vi "04_co_dela_necelistvy_pocet_period.vi"() -> ()   [LabVIEW 2019]
uses:
  <vilib>/Analysis/5stat.llb/RMS (DBL).vi
  <vilib>/measure/NI_MABase.lvlib
  <vilib>/Analysis/NI_AALPro.lvlib
panel:
  out "Spektra":T1(graph)
  out "Absolutni chyba (V)":dbl
  out "Relativni chyba (%)":dbl
  out "RMS prubehy":cluster{dbl, dbl, dbl, dbl}(graph)
  out "RMS (V)":dbl
  out "RMS (V)":dbl
  out "RMS (mat funkce) (V)":dbl format="%0.2f"
  out "RMS (mat funkce) (V)":dbl format="%0.2f"
  out "Casove prubehy":waveform(dbl)[](graph)
  out "dt (s)":dbl=0.001
  out "Vzorkovaci Frekvence (N)":dbl=1000.0
  in  "Amplituda sumu":dbl=0.9999999999999999 format="%.2p"
  in  "Faze":dbl format="%.2p"
  in  "Amplituda":dbl=10.0 format="%0.2p"
  in  "Frekvence":dbl=10.0 format="%0.2p"
  # "CELISTVY POCET PERIOD"
  # "NECELISTVY POCET PERIOD"
  # "SLEDUJTE\nJAK SE \nCHOVAJI\nJEDNOTLIVE\nVYPOCTY !"
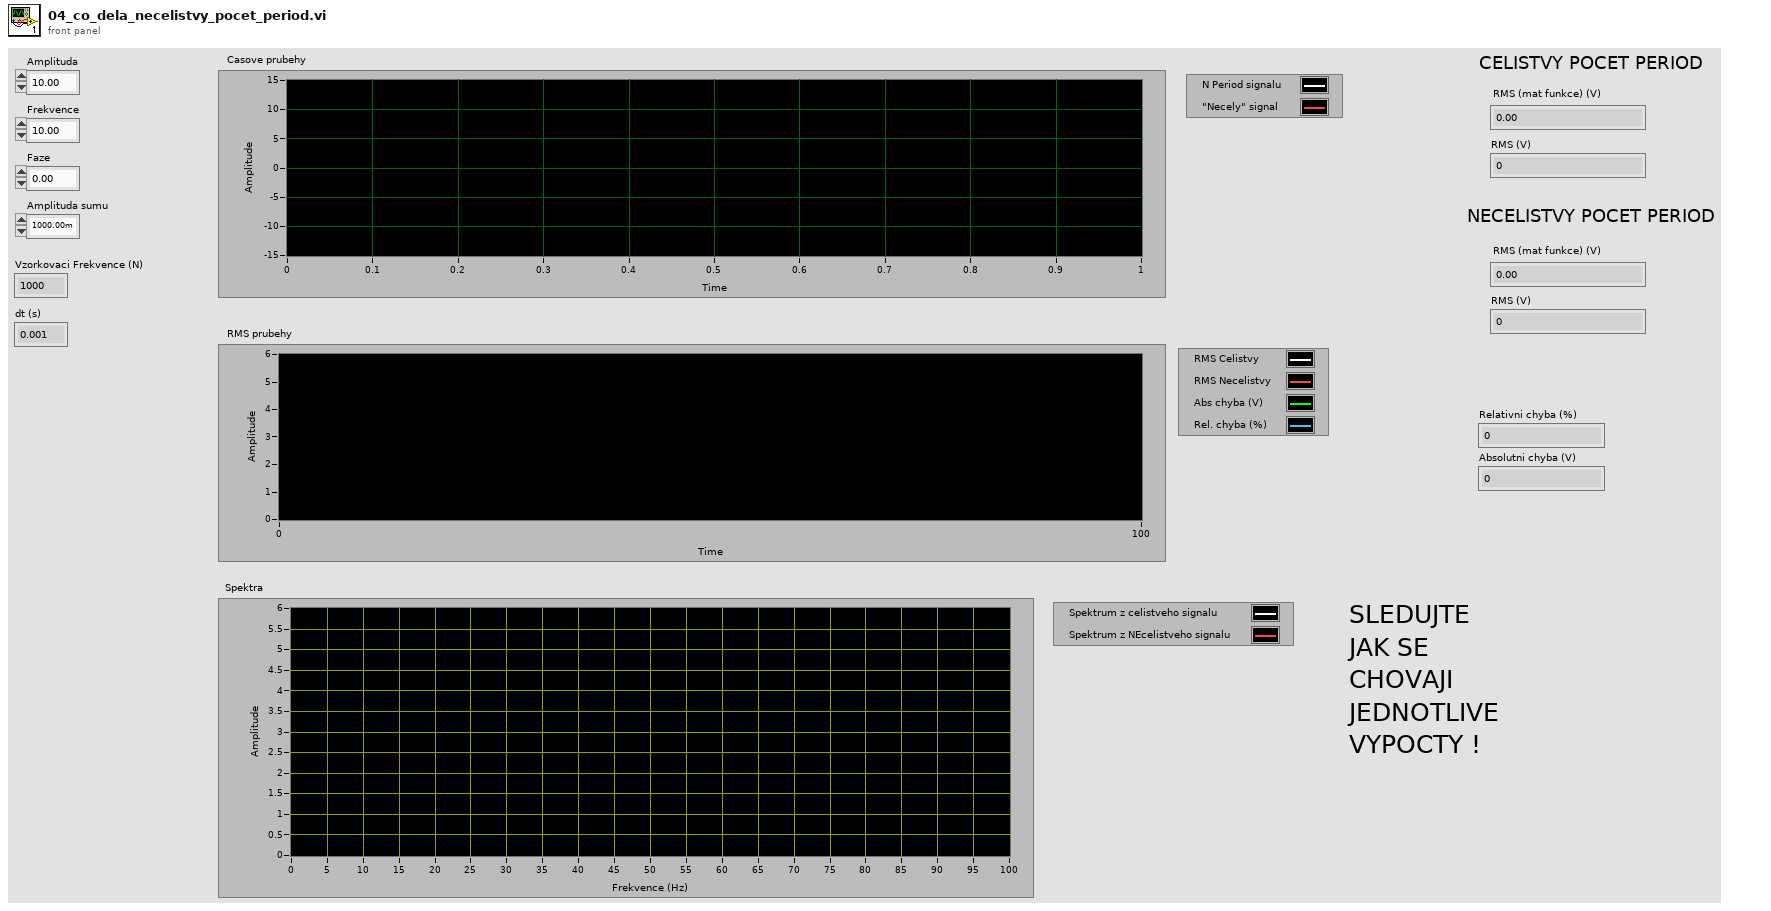
[diagram p1: front panel]
types:
  T1 = cluster{dbl[], "Amp Spectrum Mag (Vrms)":dbl[]}[]
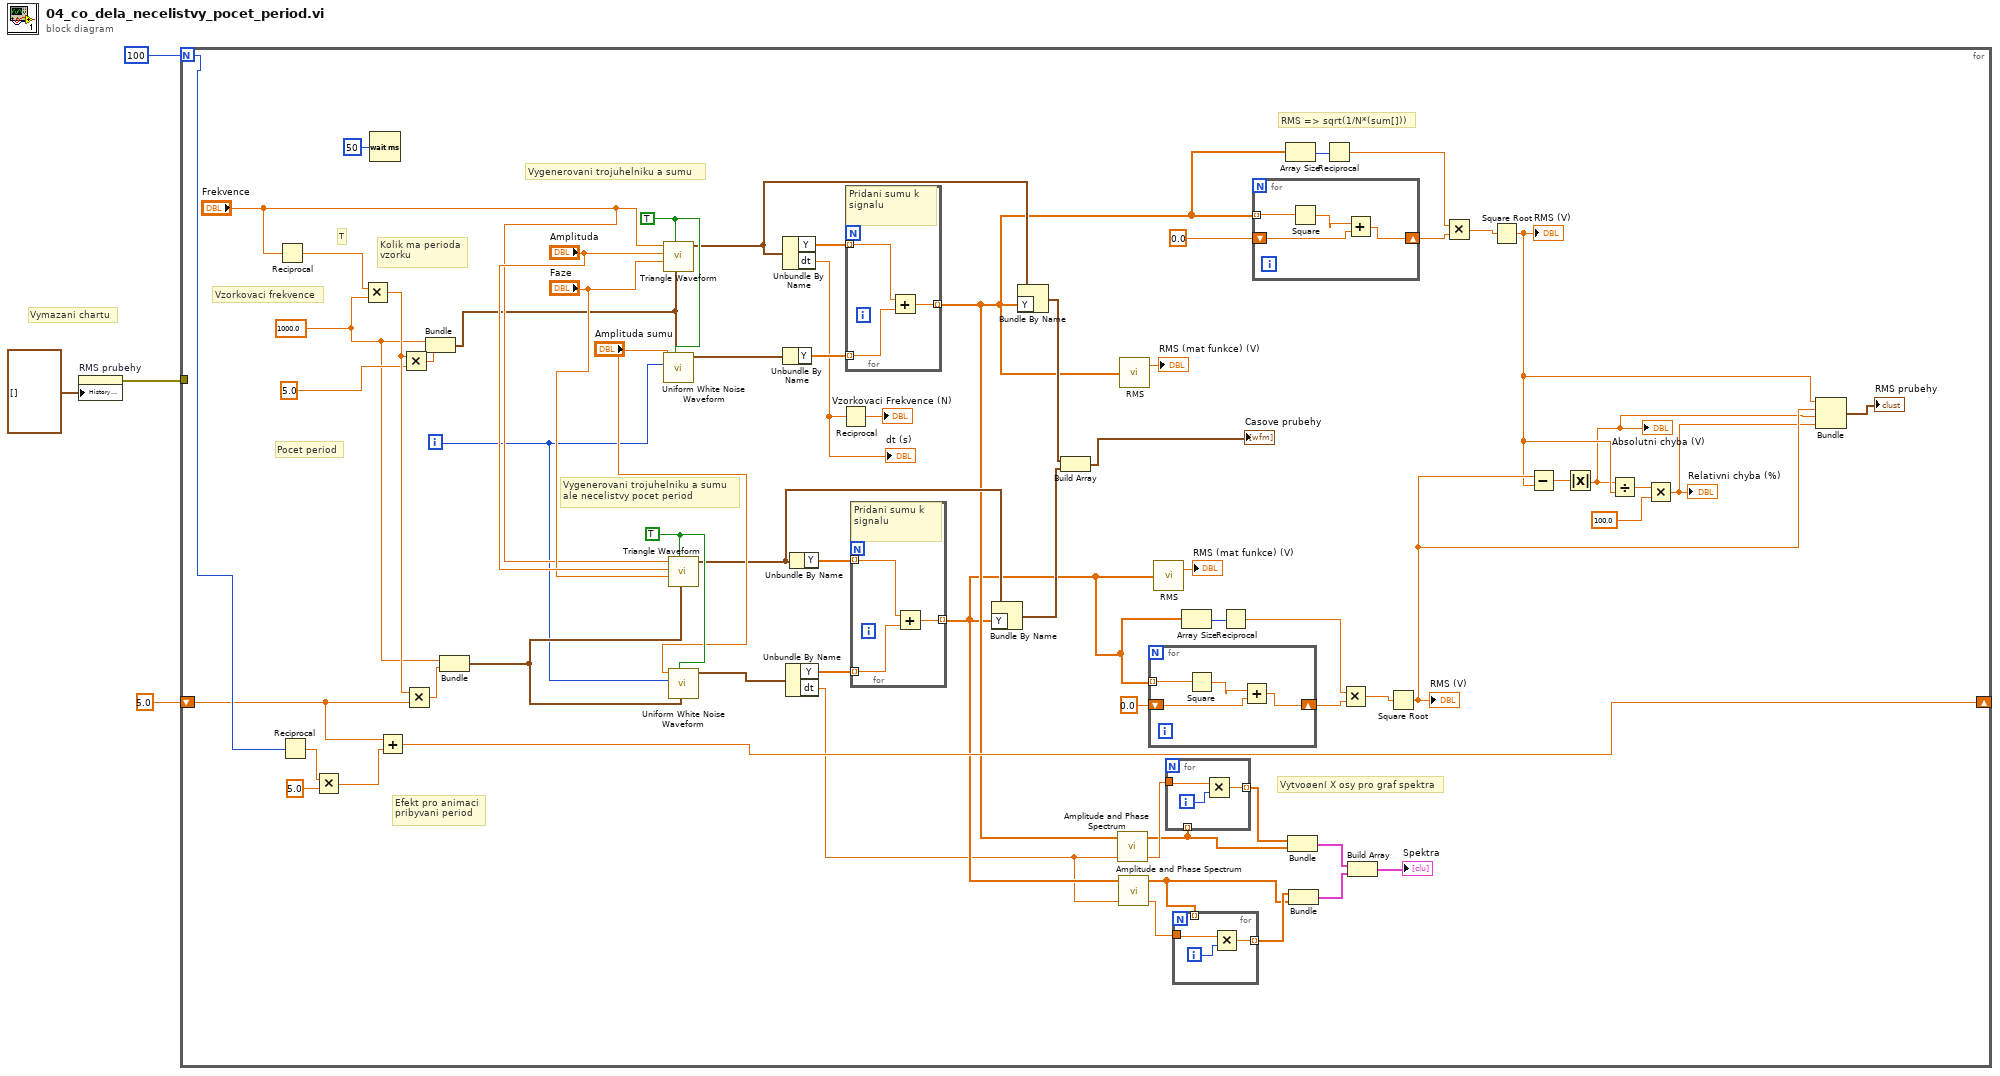
[diagram p0: block diagram]
diagram:
  # "Vymazani chartu"
  n1 = property on="RMS prubehy" class="WFChart (strict)"("History Data"=cluster{dbl, dbl, dbl, dbl}[] []) -> (error out=w2:errorcluster)  [unwired: 2 in, 1 out]
  n2 = for {
    N: 100 -> [w35]
    shift-right: [w33] -> _
    shift-left: 5.0 -> [w34]
    tunnel: w2 -> [_]
    i -> [w23]
    w24 = 1000.0 ("y")
    w62 = TRUE ("reset signal")
    w71 = TRUE ("reset signal")
    # "Vytvoøení X osy pro graf spektra"
    # "Efekt pro animaci\npribyvani period"
    # "Kolik ma perioda\nvzorku"
    # "T"
    # "Pocet period"
    # "Vzorkovaci frekvence"
    # "RMS => sqrt(1/N*(sum[]))"
    # "Vygenerovani trojuhelniku a sumu\nale necelistvy pocet period"
    # "Vygenerovani trojuhelniku a sumu"
    n3 = Reciprocal(x="Frekvence") -> (1/x=w42:dbl)
    n4 = Reciprocal(x=w35) -> (1/x=w8:dbl)
    n5 = Multiply(x=w8, y=5.0) -> (x*y=w6:dbl)
    n6 = Multiply(x=w42, y=w24) -> (x*y=w39:dbl)
    n7 = Wait (ms)(milliseconds to wait=u32 50) -> ()  [unwired: 1 out]
    n8 = Add(x=w34, y=w6) -> (x+y=w33:dbl)
    n9 = Multiply(x=w39, y=5.0) -> (x*y=w40:dbl)
    n10 = Multiply(x=w39, y=w34) -> (x*y=w38:dbl)
    n11 = Bundle("y"=w24, w40) -> (w41:cluster{"y":dbl, dbl})  [unwired: 1 in]
    n12 = Bundle("y"=w24, w38) -> (w37:cluster{"y":dbl, dbl})  [unwired: 1 in]
    n13 = call <vilib>:"Triangle Waveform.vi"("sampling info"=w41, "reset signal"=w71, "phase"="Faze", "amplitude"="Amplituda", "frequency"="Frekvence") -> ("signal out"=w58:waveform(dbl))  [unwired: 5 in, 1 out]
    n14 = call <vilib>:"Uniform White Noise Waveform.vi"("sampling info"=w41, "reset signal"=w71, "seed"=w23, "amplitude"="Amplituda sumu") -> ("signal out"=w70:waveform(dbl))  [unwired: 6 in, 1 out]
    n15 = call <vilib>:"Triangle Waveform.vi"("sampling info"=w37, "reset signal"=w62, "phase"="Faze", "amplitude"="Amplituda", "frequency"="Frekvence") -> ("signal out"=w57:waveform(dbl))  [unwired: 5 in, 1 out]
    n16 = call <vilib>:"Uniform White Noise Waveform.vi"("sampling info"=w37, "reset signal"=w62, "seed"=w23, "amplitude"="Amplituda sumu") -> ("signal out"=w63:waveform(dbl))  [unwired: 6 in, 1 out]
    n17 = Unbundle By Name(w58) -> ("Y"=w69:dbl[], "dt"=w67:dbl)
    "dt (s)" <- w67
    n18 = Unbundle By Name(w70) -> ("Y"=w68:dbl[])
    n19 = Unbundle By Name(w63) -> ("Y"=w65:dbl[], "dt"=w18:dbl)
    n20 = Unbundle By Name(w57) -> ("Y"=w64:dbl[])
    n21 = Reciprocal(x=w67) -> (1/x=→"Vzorkovaci Frekvence (N)":dbl)
    n22 = for {
      tunnel: w69 -> [w90] mode=indexing
      tunnel: w68 -> [w91] mode=indexing
      tunnel: [w89] -> w20 mode=indexing
      # "Pridani sumu k signalu"
      n23 = Add(x=w90, y=w91) -> (x+y=w89:dbl)
    }
    n24 = for {
      tunnel: w64 -> [w87] mode=indexing
      tunnel: w65 -> [w88] mode=indexing
      tunnel: [w86] -> w19 mode=indexing
      # "Pridani sumu k signalu"
      n25 = Add(x=w87, y=w88) -> (x+y=w86:dbl)
    }
    n26 = Bundle By Name(cluster=w57, "Y"=w19) -> (w56:waveform(dbl))
    n27 = Bundle By Name(cluster=w58, "Y"=w20) -> (w55:waveform(dbl))
    n28 = Build Array(w55, w56) -> (→"Casove prubehy":waveform(dbl)[])
    n29 = call <vilib>:"Amplitude and Phase Spectrum.vi"("dt"=w18, "Signal (V)"=w20) -> ("df"=w11:dbl, "Amp Spectrum Mag (Vrms)"=w10:dbl[])  [unwired: 1 in, 1 out]
    n30 = call <vilib>:"Amplitude and Phase Spectrum.vi"("dt"=w18, "Signal (V)"=w19) -> ("df"=w17:dbl, "Amp Spectrum Mag (Vrms)"=w12:dbl[])  [unwired: 1 in, 1 out]
    n31 = call-poly <vilib>:"RMS.vi"("X"=w20) -> ("rms value"=→"RMS (mat funkce) (V)":dbl)  [unwired: 1 out]
    n32 = for {
      tunnel: w19 -> [w81] mode=indexing
      shift-right: [w78] -> w44
      shift-left: 0.0 -> [w79]
      n33 = Square(x=w81) -> (x^2=w80:dbl)
      n34 = Add(x=w80, y=w79) -> (x+y=w78:dbl)
    }
    n35 = call-poly <vilib>:"RMS.vi"("X"=w19) -> ("rms value"=→"RMS (mat funkce) (V)":dbl)  [unwired: 1 out]
    n36 = for {
      tunnel: w11 -> [w74]
      tunnel: [w72] -> w9 mode=indexing
      tunnel: w10 -> [_] mode=indexing
      i -> [w73]
      n37 = Multiply(x=w74, y=w73) -> (x*y=w72:dbl)
    }
    n38 = for {
      tunnel: w17 -> [w77]
      tunnel: [w75] -> w16 mode=indexing
      tunnel: w12 -> [_] mode=indexing
      i -> [w76]
      n39 = Multiply(x=w77, y=w76) -> (x*y=w75:dbl)
    }
    n40 = Array Size(array=w19) -> (size(s)=w45:i32)
    n41 = Reciprocal(x=w45) -> (1/x=w46:dbl)
    n42 = for {
      tunnel: w20 -> [w85] mode=indexing
      shift-right: [w82] -> w51
      shift-left: 0.0 -> [w83]
      n43 = Square(x=w85) -> (x^2=w84:dbl)
      n44 = Add(x=w84, y=w83) -> (x+y=w82:dbl)
    }
    n45 = Array Size(array=w20) -> (size(s)=w50:i32)
    n46 = Bundle(w9, "Amp Spectrum Mag (Vrms)"=w10) -> (w14:cluster{dbl[], "Amp Spectrum Mag (Vrms)":dbl[]})  [unwired: 1 in]
    n47 = Bundle(w16, "Amp Spectrum Mag (Vrms)"=w12) -> (w15:cluster{dbl[], "Amp Spectrum Mag (Vrms)":dbl[]})  [unwired: 1 in]
    n48 = Reciprocal(x=w50) -> (1/x=w49:dbl)
    n49 = Multiply(x=w46, y=w44) -> (x*y=w47:dbl)
    n50 = Build Array(w14, w15) -> (→"Spektra":T1)
    n51 = Square Root(x=w47) -> (sqrt(x)=w31:dbl)
    "RMS (V)" <- w31
    n52 = Multiply(x=w49, y=w51) -> (x*y=w48:dbl)
    n53 = Square Root(x=w48) -> (sqrt(x)=w29:dbl)
    "RMS (V)" <- w29
    n54 = Subtract(x=w31, y=w29) -> (x-y=w30:dbl)
    n55 = Absolute Value(x=w30) -> (abs(x)=w26:dbl)
    "Absolutni chyba (V)" <- w26
    n56 = Divide(x=w26, y=w29) -> (x/y=w28:dbl)
    n57 = Multiply(x=w28, y=100.0) -> (x*y=w25:dbl)
    "Relativni chyba (%)" <- w25
    n58 = Bundle(w29, w31, w26, w25) -> (→"RMS prubehy":cluster{dbl, dbl, dbl, dbl})  [unwired: 1 in]
  }
